vi "Function of Position (SubVI).vi"(7 "N (Rot)":u32, 8 "n":dbl, 11 "Final Angle":dbl) -> (0 "Timestep (ms)":dbl, 2 "Current Angle":dbl, 3 "Stage Position (mm)":dbl=82.85700225830078, 4 "Angle >= Final?":bool)   [LabVIEW 2012]
uses:
  variables/GlobalUI.vi
  Rotation Mount Global.vi
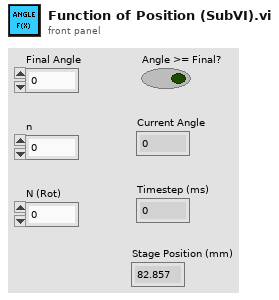
[diagram p1: front panel]
types:
  T1 = typedef "Stage Parameters.ctl" = cluster{"Scan Mode":T2, "Start position mm":dbl, "End position mm":dbl, "Velocity um/sec (continuous)":dbl, "Step size microns (discrete)":dbl, "Frames to grab (grab)":i32, "Sync Rotation with Stage":bool}
  T2 = typedef "ScanMode.ctl" = enum16{"None", "Continuous", "Point Scan (CH3 cursor)", "Point Scan Move (CH3 cursor)", "Grab", "Grab Move Stage", "Grab Move Z-stage", "Cont. Move Z-stage", "Spec Move Stage", "Spec Move Cont", "Surf Calib"}
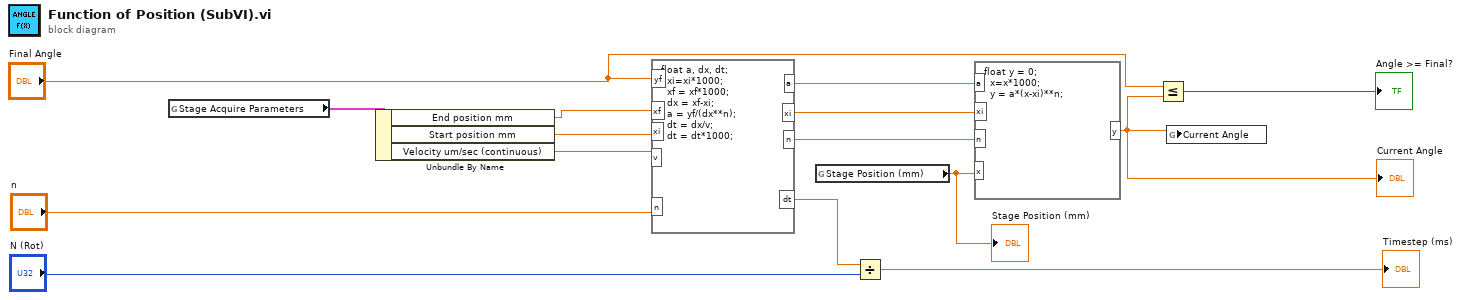
[diagram p0: block diagram]
diagram:
  n1 = global read "GlobalUI.vi" "Stage Acquire Parameters"() -> (w13:T1)
  n2 = Unbundle By Name(w13) -> ("End position mm"=w2:dbl, "Start position mm"=w1:dbl, "Velocity um/sec (continuous)"=w14:dbl)
  n3 = formula code="float a, dx, dt;\n  xi=xi*1000;\n  xf = xf*1000;\n  dx = xf-xi;\n  a = yf/(dx**n);\n  dt = dx/v;\n  dt = dt*1000;"("xf"=w2, "xi"=w1, "yf"="Final Angle", "n"="n", "v"=w14) -> ("a"=w5:dbl, "xi"=w6:dbl, "n"=w7:dbl, "dt"=w11:dbl)
  n4 = global read "GlobalUI.vi" "Stage Position (mm)"() -> (w15:dbl)
  "Stage Position (mm)" <- w15
  n5 = Divide(x=w11, y="N (Rot)") -> (x/y=→"Timestep (ms)":dbl)
  n6 = formula code="float y = 0;\n  x=x*1000;\n  y = a*(x-xi)**n;"("a"=w5, "xi"=w6, "x"=w15, "n"=w7) -> ("y"=w8:dbl)
  "Current Angle" <- w8
  n7 = Less Or Equal?(x="Final Angle", y=w8) -> (x <= y?=→"Angle >= Final?":bool)
  n8 = global write "Rotation Mount Global.vi" "Current Angle"(w8) -> ()
